vi "FGA Add Client Rec.vi"(2 "ID":u32, 3 "Network Location":T1) -> (1 "Added?":bool)   [LabVIEW 2011]
doc: "Checks the client library to see if the client has already been added. Then, if the client has not been added, adds the source ID and network location to the client library."
uses:
  UDP Lib/UDP Network Location.ctl
  Source ID Network Location Pair.ctl
  cRIO/Functional Global Variables/Actions for FG's.ctl
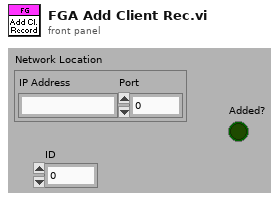
[diagram p1: front panel]
types:
  T1 = typedef "UDP Network Location.ctl" = cluster{"IP Address":string, "Port":u16}
  T2 = typedef "Source ID Network Location Pair.ctl" = cluster{"ID":u32, "Network Location":T1}
  T3 = typedef "Actions for FG's.ctl" = enum16{"Read", "Write"}
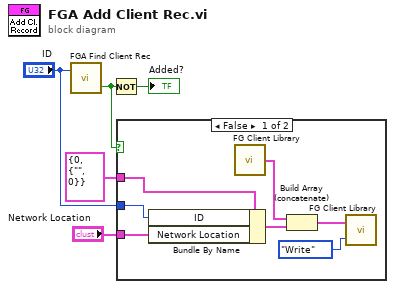
[diagram p0: block diagram]
diagram:
  n1 = call "FGA Find Client Rec.vi"("Source ID"="ID") -> ("Record Exists?"=w2:bool)  [unwired: 1 in, 1 out]
  n2 = Not(x=w2) -> (.not. x?=→"Added?":bool)
  n3 = case shown="False" w2 {
    tunnel: T2 {"ID"=0, "Network Location"={"IP Address"="", "Port"=0}} ("Record out") -> [w12 _]
    tunnel: "ID" -> [w11 _]
    tunnel: "Network Location" -> [w10 _]
    frame False {
      n4 = Bundle By Name(cluster=w12, "ID"=w11, "Network Location"=w10) -> (w8:T2)
      n5 = call "FG Client Library.vi"() -> ("Client Records out"=w9:T2[])  [unwired: 2 in]
      n6 = Build Array (concatenate)(w9, w8) -> (w7:T2[])
      n7 = call "FG Client Library.vi"("FG Action (Read)"=Actions_for_FG's."Write", "Client Records in"=w7) -> ()  [unwired: 1 out]
    }
    frame True {
    }
  }
